vi "Increment Build.vi"(1 "Current Version":string) -> (2 "next version":string)   [LabVIEW 2025, in "App-Builder Library.lvlib" / "Builder.lvclass"]
uses:
  Builder.lvclass
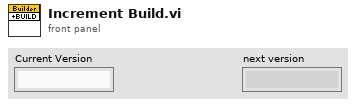
[diagram p1: front panel]
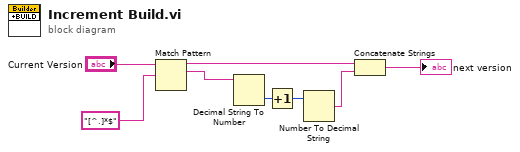
[diagram p0: block diagram]
diagram:
  n1 = Match Pattern(string="Current Version", regular expression="[^.]*$") -> (before substring=w6:string, match substring=w2:string)  [unwired: 1 in, 2 out]
  n2 = Decimal String To Number(string=w2) -> (number=w5:i32)  [unwired: 2 in, 1 out]
  n3 = Increment(x=w5) -> (x+1=w4:i32)
  n4 = Number To Decimal String(number=w4) -> (decimal integer string=w3:string)  [unwired: 1 in]
  n5 = Concatenate Strings(w6, w3) -> (→"next version":string)
